vi "GetData.vi"(11 "Sig_DA in":refnum<class "DA.lvclass">) -> (2 "data":T1)   [LabVIEW 2019, in "DA.lvclass"]
uses:
  DA.lvclass
  TypeDef/bool_data.ctl
  DA.lvclass/DA.ctl
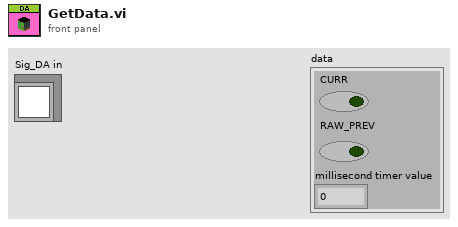
[diagram p1: front panel]
types:
  T1 = typedef "bool_data.ctl" = cluster{"CURR":bool, "RAW_PREV":bool, "millisecond timer value":u32}
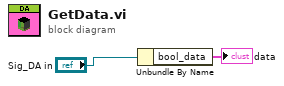
[diagram p0: block diagram]
diagram:
  n1 = Unbundle By Name("Sig_DA in") -> ("bool_data"=→"data":T1)
